vi "FlashingAnLED_Myrio.vi"   [LabVIEW 2012]
types:
  T1 = typedef "BotSpeak_Control.ctl" = cluster{"Address":string, "Reply EOF":string, "Hardware":string, "Retries":i8, "Timeout":i32}
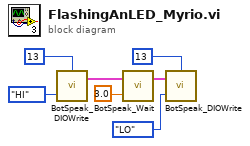
[diagram p0: block diagram]
diagram:
  n1 = call <userlib>:"BotSpeak_DIOWrite.vi"("State"=enum32{"LO", "HI"}."HI", "DIO Line"=u32 13) -> ("Bot Settings"=w6:T1)  [unwired: 1 in, 1 out]
  n2 = call <userlib>:"BotSpeak_Wait.vi"("Wait (sec)"=3.0, "Bot Settings"=w6) -> ("Bot Settings"=w3:T1)  [unwired: 1 in]
  n3 = call <userlib>:"BotSpeak_DIOWrite.vi"("State"=enum32{"LO", "HI"}."LO", "Bot Settings"=w3, "DIO Line"=u32 13) -> ()  [unwired: 2 out]
